vi "chaos crest cu get channel.vi"(6 "maxsize":i32, 7 "value":string, 9 "channame":string, 10 "cuname":string, 11 "handleConnection":u32) -> (3 "timestamp":u32, 5 "value out":string)   [LabVIEW 2014, in "libcommon-crest.lvlib"]
doc: "uint64_t chaos_crest_cu_get_channel(chaos_crest_handle_t h,const char*cuname,const char*channame,char*output,int maxsize);"
uses:
  libcommon-crest.lvlib
  chaos-i686-dynamic-release/lib/libcommon-crest.so
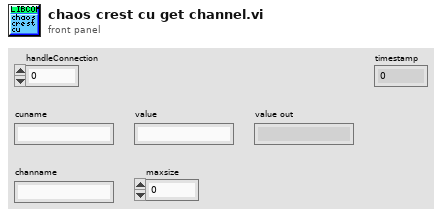
[diagram p1: front panel]
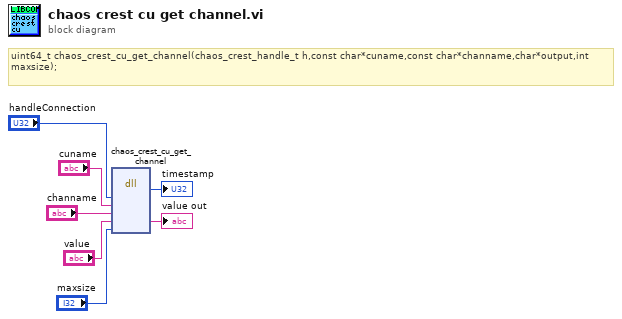
[diagram p0: block diagram]
diagram:
  # "uint64_t chaos_crest_cu_get_channel(chaos_crest_handle_t h,const char*cuname,const char*channame,char*output,int maxsize);"
  n1 = dll-call lib="home/chaos/chaos_bundle/chaos-i686-dynamic-release/lib/libcommon-crest.*" fn="chaos_crest_cu_get_channel"("handleConnection"="handleConnection", "cuname"="cuname", "channame"="channame", "value"="value", "maxsize"="maxsize") -> (→"timestamp":u32, "value"=→"value out":string)  [unwired: 7 in, 2 out]
